vi "Button Toggle Arrays.vi"(11 "Joystick_SEN_Buttons":bool[](array[boolean])) -> (1 "Falling Edge Outputs Out":bool[](array[boolean]), 2 "Rizing Edge Outputs Out":bool[](array[boolean]), 3 "Toggle Outputs Out":bool[](array[boolean]))   [LabVIEW 2017]
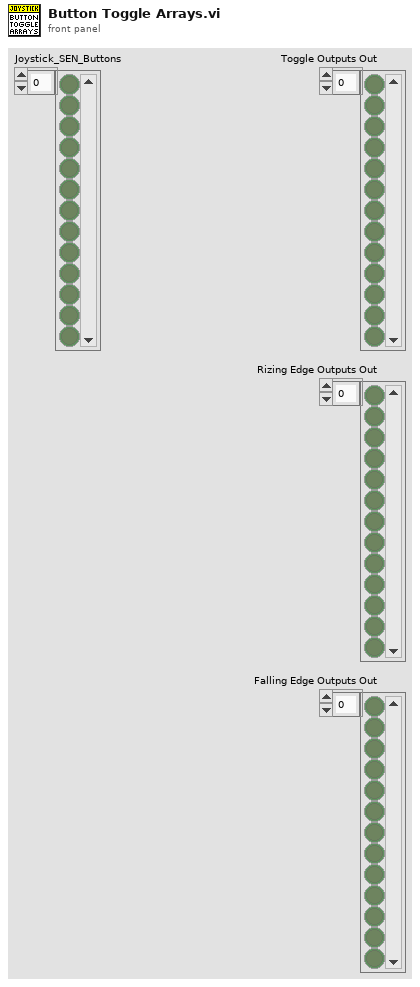
[diagram p1: front panel]
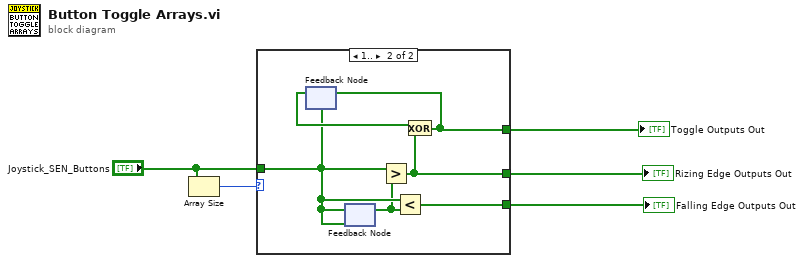
[diagram p0: block diagram]
diagram:
  n1 = Array Size(array="Joystick_SEN_Buttons") -> (size(s)=w3:i32)
  n2 = case shown="1.." w3 {
    tunnel: [w6 w12] -> w5
    tunnel: "Joystick_SEN_Buttons" -> [w6 w9]
    tunnel: [w6 w10] -> w2
    tunnel: [w6 w7] -> w1
    frame ..0 {
    }
    frame 1.. {
      n3 = feedback #1(w9) -> (w11:bool[])
      n4 = feedback #2(w9) -> (w8:bool[])
      n5 = feedback-in #2(w9) -> ()
      n6 = Greater?(x=w9, y=w8) -> (0:w10:bool[])
      n7 = Less?(x=w9, y=w8) -> (x < y?=w7:bool[])
      n8 = Exclusive Or(1:w10, 2:w11) -> (0:w12:bool[])
      n9 = feedback-in #1(w12) -> ()
    }
  }
  "Toggle Outputs Out" <- w5
  "Rizing Edge Outputs Out" <- w2
  "Falling Edge Outputs Out" <- w1
